vi "Add.vi"(10 "B":dbl, 11 "x":dbl) -> (2 "x+B":dbl)   [LabVIEW 2020]
panel:
  out "XY Graph":cluster{"X":dbl, "Y":dbl}[](graph)
  # "Hello world"
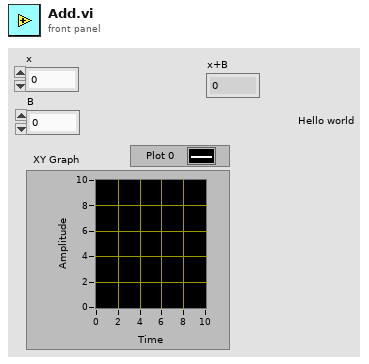
[diagram p1: front panel]
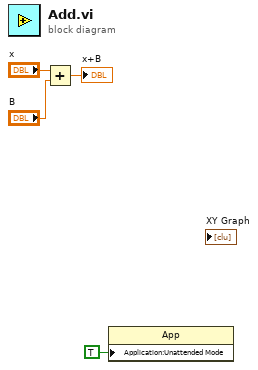
[diagram p0: block diagram]
diagram:
  n1 = Add(x="x", y="B") -> (x+y=→"x+B":dbl)
  n2 = property class="App"("Application:Unattended Mode"=TRUE) -> ()  [unwired: 2 in, 2 out]
